vi "constant--support folder name.vi"() -> (0 "Name of support folder":string)   [LabVIEW 2020, in "main.lvlib"]
uses:
  main.lvlib
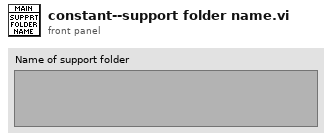
[diagram p1: front panel]
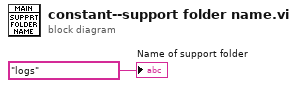
[diagram p0: block diagram]
diagram:
  "Name of support folder" <- "logs" ("Support Folder name")
